vi "总磷总氮测量流程.vi"(8 "启动参数":cluster{"总磷":bool, "总氮":bool}={"总磷"=TRUE, "总氮"=TRUE}, 9 "总氮量程模式":T1, 10 "总磷量程模式":T1, 11 "参数":T2={"站号"=1, "量程切换"=enum."AUTO", "控制命令"=enum."启动测量", "模式设置"=enum."待机", "测量间隔"=0} {"站号" items=["总磷"=1, "总氮"=2]}) -> ()   [LabVIEW 2016, in "斯坦道总磷总氮.lvlib"]
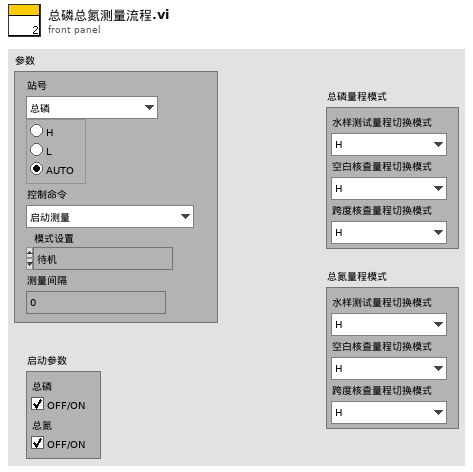
[diagram p1: front panel]
types:
  T1 = cluster{"水样测试量程切换模式":enum16{"H", "L", "AUTO"}, "空白核查量程切换模式":enum16{"H", "L", "AUTO"}, "跨度核查量程切换模式":enum16{"H", "L", "AUTO"}}
  T2 = cluster{"站号":u16, "量程切换":enum32{"H", "L", "AUTO"}, "控制命令":enum16{"启动测量", "标样核查", "零点核查", "跨度核查", "空白测试", "平行样测试", "加标回收", "空白校准", "标样校准", "初始化（清洗）", "停止测试", "仪器重启", "校时", "模式设置", "测量间隔设置"}, "模式设置":enum16{"待机", "连续模式", "周期模式", "定点模式", "受控模式", "手动模式"}, "测量间隔":u16}
  T3 = enum16{"初始化", "通电", "参数1启动", "等待参数1测试完成", "参数1测试完成", "参数1存储数据", "参数2启动", "等待参数2测试完成", "参数2测试完成", "参数2存储数据", "断电", "结束"}
  T4 = cluster{"运行模式":enum16{"维护模式", "常规模式", "应急模式", "质控模式"}, "质控频次":enum16{"关闭", "每天", "星期一", "星期二", "星期三", "星期四", "星期五", "星期六", "星期日"}, "空白核查时间":u16, "跨度核查时间":u16, "24H周期设置":bool[]}
  T5 = cluster{"时间标识":timestamp, "设备":string, "日志信息":string, "流程参数":string}
  T6 = cluster{"时间标识":timestamp, "监测值":sgl, "单位":u16, "数据标识":string, "因子编码":u32, "标样参考值":sgl, "F0":sgl, "F1":sgl, "F2":sgl, "F3":sgl, "F4":sgl, "F5":sgl, "F6":sgl, "F7":sgl, "X":sgl, "温度":sgl, "湿度":sgl, "量程标识":string}
  T7 = enum16{"维护数据", "水样测试", "标样核查", "零点核查", "跨度核查", "空白测试", "平行样测试", "加标回收", "空白校准", "标样校准", "初始化（清洗）"}
  T8 = enum16{"启动测量", "标样核查", "零点核查", "跨度核查", "空白测试", "平行样测试", "加标回收", "空白校准", "标样校准", "初始化（清洗）", "停止测试", "仪器重启", "校时", "模式设置", "测量间隔设置"}
  T9 = cluster{"系统时间":timestamp, "工作状态":enum16{"空闲", "水样测试", "标样核查", "零点核查", "跨度核查", "空白测试", "平行样测试", "加标回收", "空白校准", "标样校准", "初始化（清洗）"}, "测量模式":enum16{"待机", "连续模式", "周期模式", "定点模式", "受控模式", "手动模式"}, "告警代码":enum16{"无告警", "缺试剂告警", "缺水样告警", "缺蒸馏水告警", "缺标液告警", "仪表漏液告警", "标定异常告警", "超量程告警", "加热异常", "低试剂预警", "超上限告警", "超下限告警", "仪表内部其他异常", "滴定异常告警", "电极异常告警", "量程切换告警", "参数设置告警", "PH电极电位异常", "电导率电极异常", "浊度光度异常", "溶解氧电极异常", "溶解氧光强异常", "温度异常告警", "PH异常告警", "溶解氧异常告警", "电导率异常告警", "浊度异常告警", "叶绿素异常告警", "藻密度异常告警", "蓝绿藻异常告警", "ORP异常告警", "氨氮异常告警", "清洁刷异常告警", "SD卡异常告警", "蓝牙异常告警", "Wifi异常告警", "流程异常告警"}, "故障代码":enum16{"无故障", "电机故障", "温度故障", "通讯故障", "滴定故障"}, "日志代码":u16, "软件版本":u16, "F0":sgl, "F1":sgl, "F2":sgl, "F3":sgl, "T":sgl, "H":sgl, "id":u16, "flowid":u16, "量程":u16, "总磷控温温度1":sgl, "营养盐控温温度2":sgl, "ADC":sgl}
  T10 = enum16{"空闲", "水样测试", "标样核查", "零点核查", "跨度核查", "空白测试", "平行样测试", "加标回收", "空白校准", "标样校准", "初始化（清洗）"}
  T11 = cluster{"因子编码":u32, "单位":u16, "标样参考值":sgl, "水样数据时间":timestamp, "水样实测值":sgl, "水样数据标识":string, "标样数据时间":timestamp, "标样实测值":sgl, "标样数据标识":string, "空白数据时间":timestamp, "空白实测值":sgl, "空白数据标识":string, "零点核查数据时间":timestamp, "零点核查实测值":sgl, "零点核查数据标识":string, "跨度核查数据时间":timestamp, "跨度核查实测值":sgl, "跨度核查数据标识":string, "加标回收数据时间":timestamp, "加标回收实测值":sgl, "加标回收数据标识":string, "平行样数据时间":timestamp, "平行样实测值":sgl, "平行样数据标识":string, "F0":sgl, "F1":sgl, "F2":sgl, "F3":sgl, "F4":sgl, "F5":sgl, "F6":sgl, "F7":sgl, "温度":sgl, "湿度":sgl, "X值":sgl}
  T12 = cluster{"总磷跨度值":dbl, "总磷零点标准液浓度":dbl, "总磷跨度标准液浓度":dbl, "总磷标准液标准浓度":dbl, "总氮跨度值":dbl, "总氮零点标准液浓度":dbl, "总氮跨度标准液浓度":dbl, "总氮标准液标准浓度":dbl}
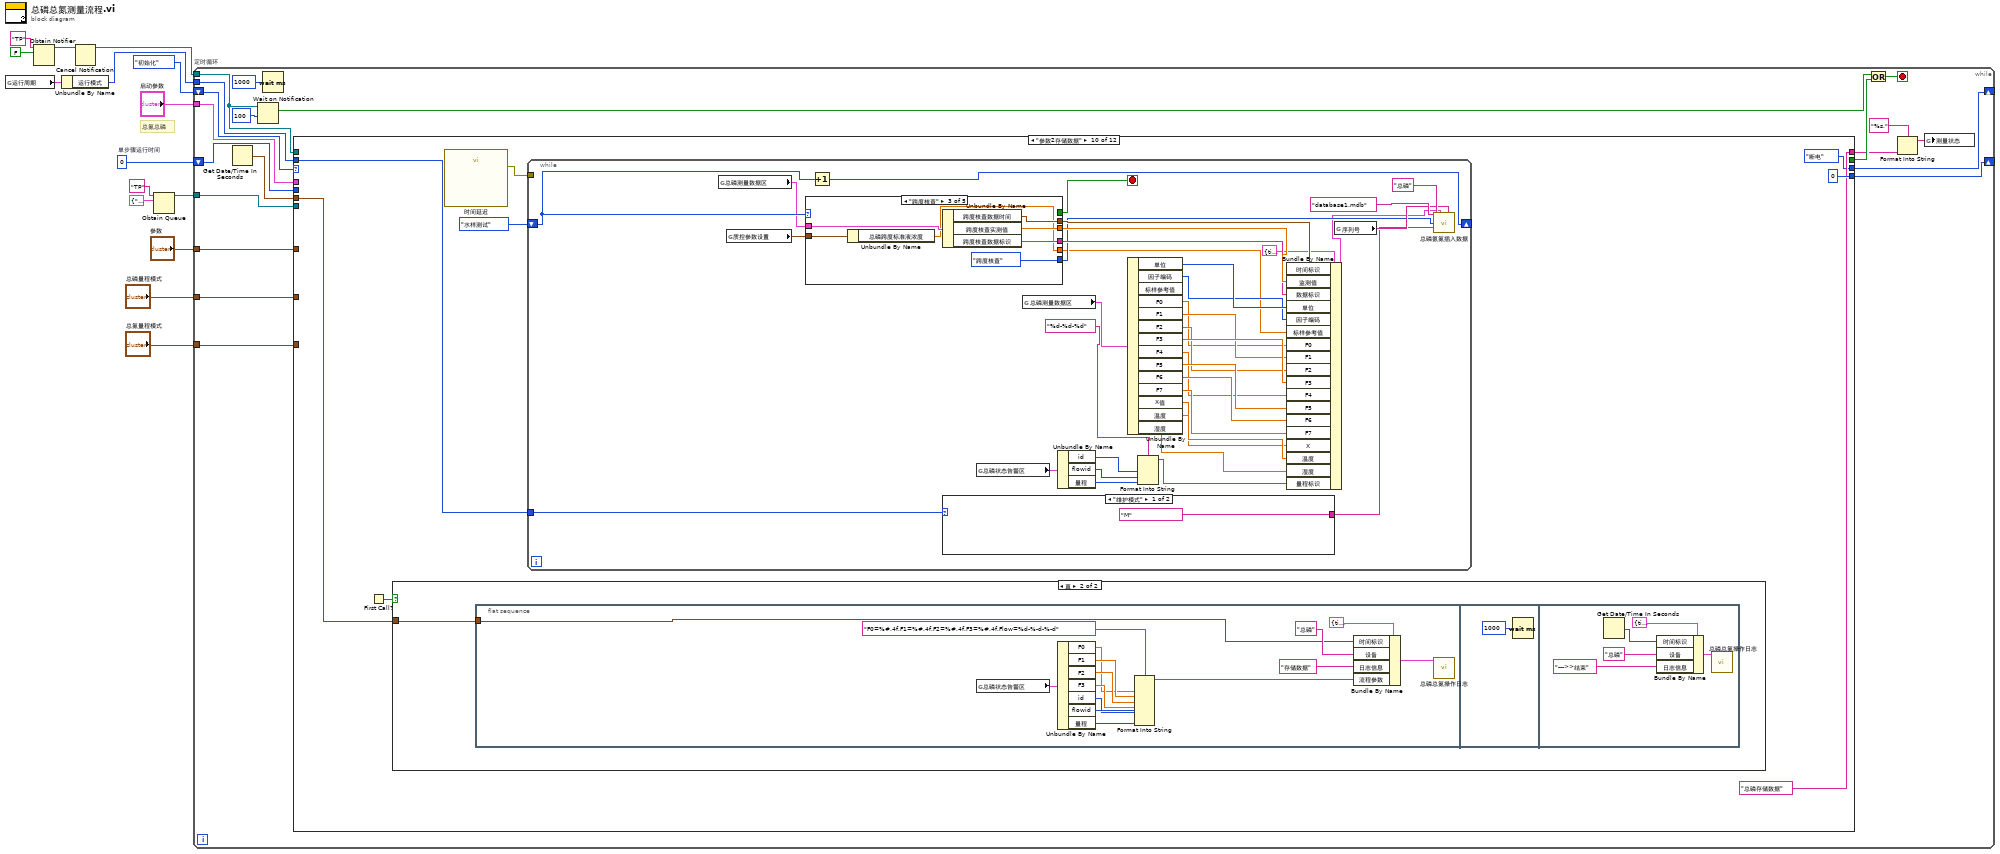
[diagram p0: block diagram]
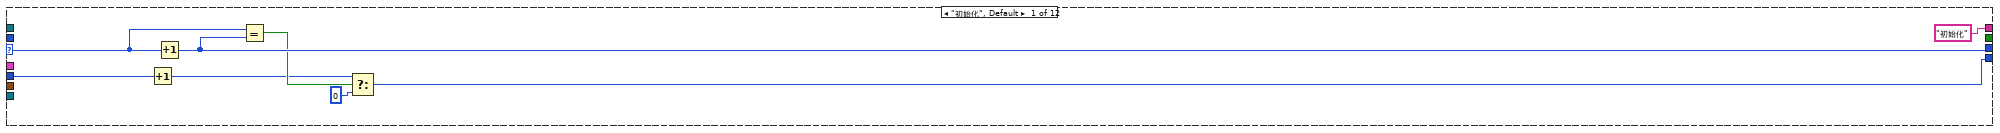
[diagram p2: hidden frame]
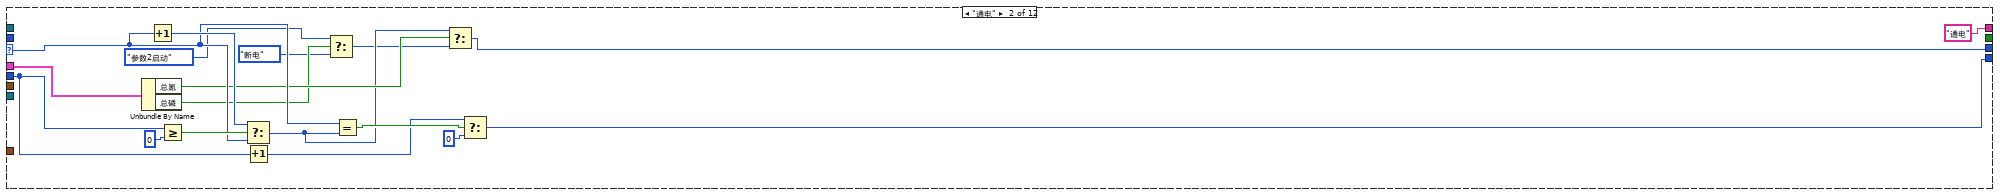
[diagram p3: hidden frame]
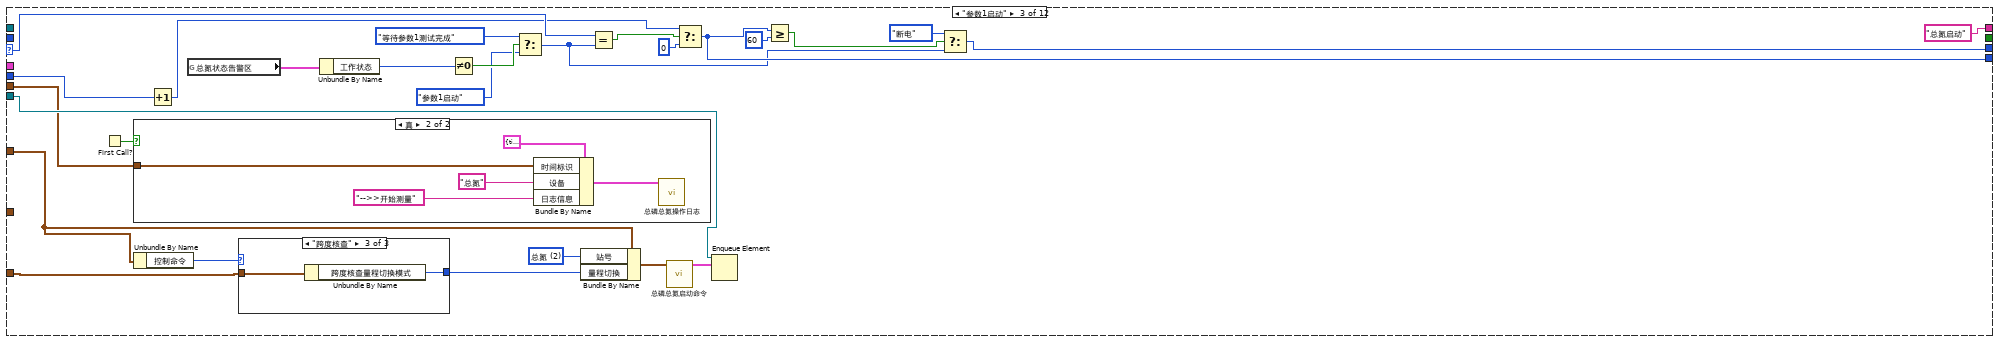
[diagram p4: hidden frame]
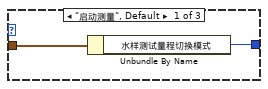
[diagram p5: hidden frame]
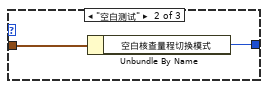
[diagram p6: hidden frame]
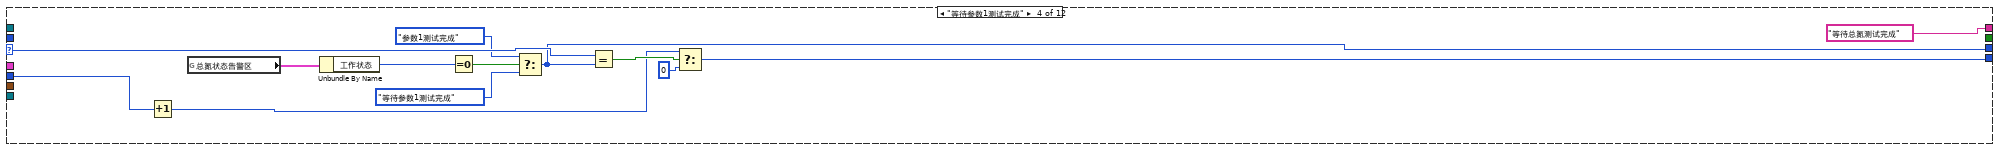
[diagram p8: hidden frame]
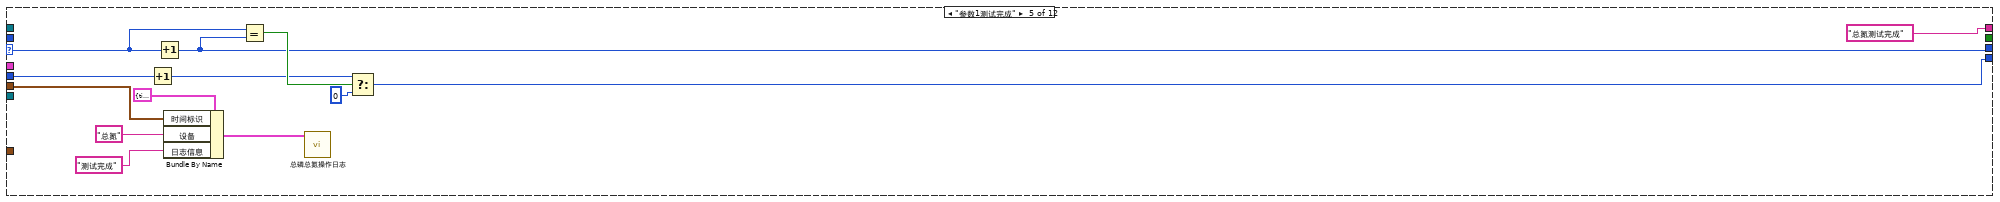
[diagram p9: hidden frame]
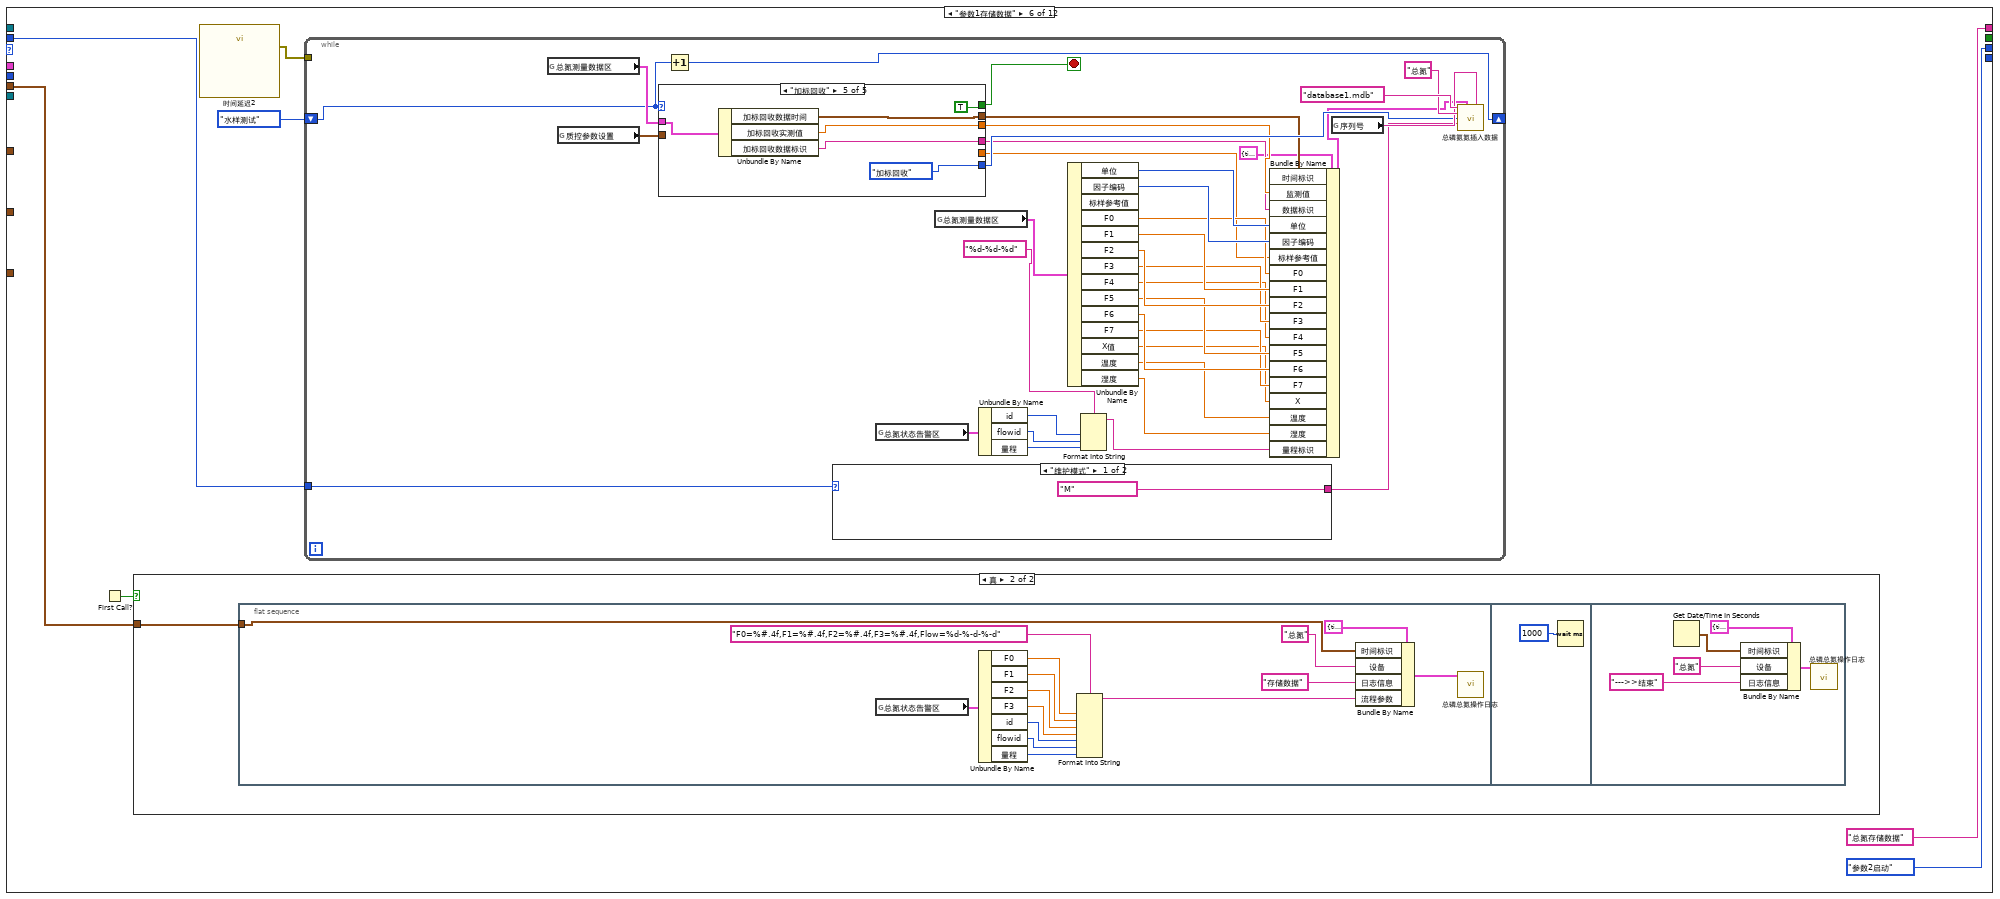
[diagram p10: hidden frame]
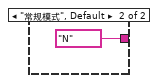
[diagram p11: hidden frame]
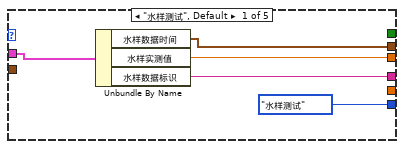
[diagram p12: hidden frame]
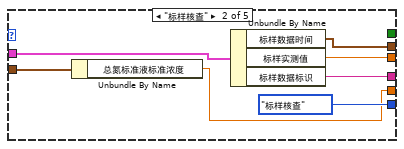
[diagram p13: hidden frame]
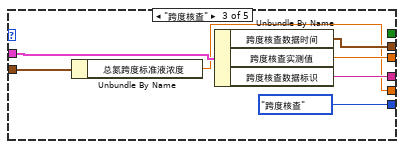
[diagram p14: hidden frame]
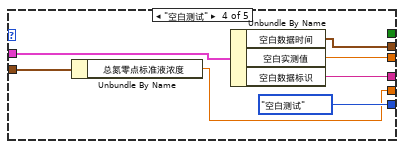
[diagram p15: hidden frame]
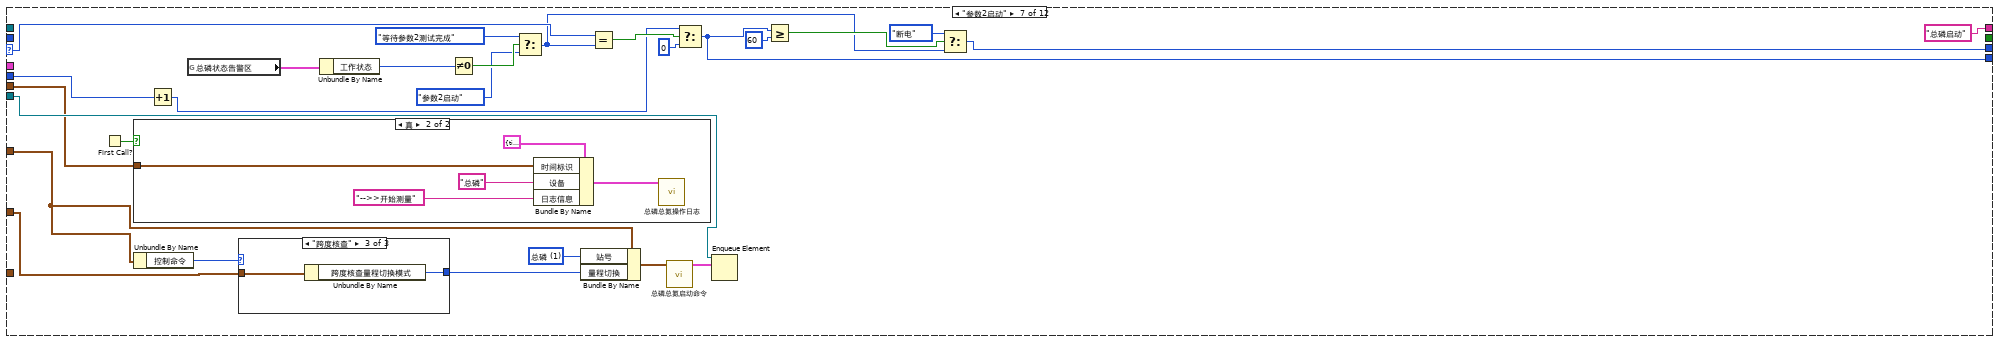
[diagram p17: hidden frame]
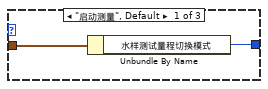
[diagram p18: hidden frame]
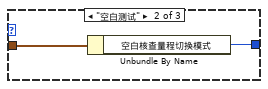
[diagram p19: hidden frame]
diagram:
  w11 = 0  # 单步骤运行时间
  # "总氮总磷"
  n1 = global read "总磷总氮断电保存全局变量.vi" "运行周期"() -> (w2:T4)
  n2 = Obtain Notifier(name (unnamed)="TP" ("名称（未命名）"), notification data type=FALSE) -> (notifier out=w8:refnum<notifier>)  [unwired: 2 in, 2 out]
  n3 = Unbundle By Name(w2) -> ("运行模式"=w1:enum16{"维护模式", "常规模式", "应急模式", "质控模式"})
  n4 = Cancel Notification(0:w8) -> (8:w7:refnum<notifier>)  [unwired: 1 in, 2 out]
  n5 = Obtain Queue(name (unnamed)="TP" ("名称（未命名）"), element data type=cluster{"命令":string, "data":variant} {"命令"="", "data"=variant}) -> (queue out=w12:refnum<queue>)  [unwired: 3 in, 2 out]
  n6 = while "定时循环" {
    shift-right: [w34] -> _
    shift-left: T3."初始化" ("枚举") -> [w35]
    tunnel: w12 -> [w33]
    shift-right: [w31] -> _
    shift-left: w11 -> [w32]
    tunnel: w7 -> [w30]
    tunnel: "参数" -> [w25]
    tunnel: "总氮量程模式" -> [w20]
    tunnel: "总磷量程模式" -> [w18]
    tunnel: "启动参数" -> [w17]
    tunnel: w1 -> [w16]
    stop <- w26 stop-if-true
    n7 = Get Date/Time In Seconds() -> (seconds since 1Jan1904=w23:timestamp)
    n8 = Wait on Notification(notifier=w30, timeout in ms (-1)=100 ("超时毫秒(-1)")) -> (notification=w27:bool)  [unwired: 2 in, 3 out]
    n9 = Wait (ms)(milliseconds to wait=u32 1000 ("等待时间（毫秒）")) -> ()  [unwired: 1 out]
    n10 = case shown="\"参数2存储数据\"" w35 {
      selector: w35 -> [w41 w55 w83 w107 w122 _ w241 w269 w285 _ w396 _]
      tunnel: [_ _ _ _ _ _ _ _ _ _ _ TRUE] -> w28
      tunnel: [w42 w48 w62 w106 w121 T3."参数2启动" ("枚举") w227 w267 w283 T3."断电" ("枚举") w395 T3."结束" ("枚举")] -> w34
      tunnel: w33 -> [_ _ w88 _ _ _ w249 _ _ _ _ w403]
      tunnel: w32 -> [w43 w56 w84 w109 w123 _ w242 w270 w286 _ w398 _]
      tunnel: [w39 w57 w67 w108 w124 _ w228 w268 w284 0 ("t") w397 0 ("t")] -> w31
      tunnel: w30 -> [_ _ _ _ _ _ _ _ _ _ _ w402]
      tunnel: w25 -> [_ _ w71 _ _ _ w235 _ _ _ _ _]
      tunnel: w23 -> [_ _ w76 _ w114 w132 w240 _ w278 w296 _ _]
      tunnel: ["初始化" ("输入 1") "通电" ("输入 1") "总氮启动" ("输入 1") "等待总氮测试完成" ("输入 1") "总氮测试完成" ("输入 1") "总氮存储数据" ("输入 1") "总磷启动" ("输入 1") "等待总磷测试完成" ("输入 1") "总磷测试完成" ("输入 1") "总磷存储数据" ("输入 1") "断电" ("输入 1") "结束" ("输入 1")] -> w21
      tunnel: w20 -> [_ _ w69 _ _ _ _ _ _ _ _ _]
      tunnel: w18 -> [_ _ _ _ _ _ w226 _ _ _ _ _]
      tunnel: w17 -> [_ w51 _ _ _ _ _ _ _ _ _ _]
      tunnel: w16 -> [_ _ _ _ _ w126 _ _ _ w290 _ _]
      frame "初始化", Default {
        n11 = Increment(x=w43) -> (x+1=w37:i32)
        n12 = Increment(x=w41) -> (x+1=w42:T3)
        n13 = Equal?(x=w41, y=w42) -> (x = y?=w40:bool)
        n14 = Select(t=w37, s=w40, f=0 ("t")) -> (s? t:f=w39:i32)
      }
      frame "通电" {
        n15 = Unbundle By Name(w51) -> ("总氮"=w50:bool, "总磷"=w47:bool)
        n16 = Increment(x=w55) -> (x+1=w59:T3)
        n17 = Greater Or Equal?(x=w56, y=0) -> (x >= y?=w60:bool)
        n18 = Select(t=w59, s=w60, f=w55) -> (s? t:f=w49:T3)
        n19 = Increment(x=w56) -> (x+1=w54:i32)
        n20 = Select(t=T3."参数2启动" ("枚举"), s=w47, f=T3."断电" ("枚举")) -> (s? t:f=w44:T3)
        n21 = Equal?(x=w55, y=w49) -> (x = y?=w58:bool)
        n22 = Select(t=w49, s=w50, f=w44) -> (s? t:f=w48:T3)
        n23 = Select(t=w54, s=w58, f=0 ("t")) -> (s? t:f=w57:i32)
      }
      frame "参数1启动" {
        w78 = u16 2 items=["总磷"=1, "总氮"=2, "氨氮"=3] ("站号")
        n24 = First Call?() -> (First Call?: T/F=w75:bool)
        n25 = case shown="真" w75 {
          tunnel: w76 -> [_ w95]
          frame False {
          }
          frame True {
            n26 = Bundle By Name(cluster=T5 {"时间标识"=timestamp(0 s since 1904-01-01), "设备"="", "日志信息"="", "流程参数"=""} ("data in"), "时间标识"=w95, "设备"="总氮", "日志信息"="-->>开始测量") -> (w99:T5)
            n27 = call "总磷总氮操作日志.vi"("data in"=w99) -> ()  [unwired: 11 in]
          }
        }
        n28 = Unbundle By Name(w71) -> ("控制命令"=w70:T8)
        n29 = Increment(x=w84) -> (x+1=w81:i32)
        n30 = global read "VAR总磷总氮全局变量.vi" "总氮状态告警区"() -> (w77:T9)
        n31 = case shown="\"跨度核查\"" w70 {
          tunnel: w69 -> [w90 w92 w94]
          tunnel: [w89 w91 w93] -> w68
          frame "启动测量", Default {
            n32 = Unbundle By Name(w90) -> ("水样测试量程切换模式"=w89:enum16{"H", "L", "AUTO"})
          }
          frame "空白测试" {
            n33 = Unbundle By Name(w92) -> ("空白核查量程切换模式"=w91:enum16{"H", "L", "AUTO"})
          }
          frame "跨度核查" {
            n34 = Unbundle By Name(w94) -> ("跨度核查量程切换模式"=w93:enum16{"H", "L", "AUTO"})
          }
        }
        n35 = Unbundle By Name(w77) -> ("工作状态"=w87:T10)
        n36 = Not Equal To 0?(x=w87) -> (x != 0?=w86:bool)
        n37 = Select(t=T3."等待参数1测试完成" ("枚举"), s=w86, f=T3."参数1启动" ("枚举")) -> (s? t:f=w64:T3)
        n38 = Bundle By Name(cluster=w71, "站号"=w78, "量程切换"=w68) -> (w79:T2)
        n39 = Equal?(x=w83, y=w64) -> (x = y?=w85:bool)
        n40 = call "总磷总氮启动命令.vi"("参数"=w79) -> ("启动命令"=w80:cluster{"命令":string, "data":variant})  [unwired: 10 in]
        n41 = Select(t=w81, s=w85, f=0 ("t")) -> (s? t:f=w67:i32)
        n42 = Enqueue Element(queue=w88, element=w80) -> ()  [unwired: 2 in, 3 out]
        n43 = Greater Or Equal?(x=w67, y=60) -> (x >= y?=w65:bool)
        n44 = Select(t=T3."断电" ("枚举"), s=w65, f=w64) -> (s? t:f=w62:T3)
      }
      frame "等待参数1测试完成" {
        n45 = Increment(x=w109) -> (x+1=w104:i32)
        n46 = global read "VAR总磷总氮全局变量.vi" "总氮状态告警区"() -> (w103:T9)
        n47 = Unbundle By Name(w103) -> ("工作状态"=w112:T10)
        n48 = Equal To 0?(x=w112) -> (x = 0?=w111:bool)
        n49 = Select(t=T3."参数1测试完成" ("枚举"), s=w111, f=T3."等待参数1测试完成" ("枚举")) -> (s? t:f=w106:T3)
        n50 = Equal?(x=w107, y=w106) -> (x = y?=w110:bool)
        n51 = Select(t=w104, s=w110, f=0 ("t")) -> (s? t:f=w108:i32)
      }
      frame "参数1测试完成" {
        n52 = Increment(x=w123) -> (x+1=w119:i32)
        n53 = Increment(x=w122) -> (x+1=w121:T3)
        n54 = Bundle By Name(cluster=T5 {"时间标识"=timestamp(0 s since 1904-01-01), "设备"="", "日志信息"="", "流程参数"=""} ("data in"), "时间标识"=w114, "设备"="总氮", "日志信息"="测试完成") -> (w118:T5)
        n55 = Equal?(x=w122, y=w121) -> (x = y?=w125:bool)
        n56 = call "总磷总氮操作日志.vi"("data in"=w118) -> ()  [unwired: 11 in]
        n57 = Select(t=w119, s=w125, f=0 ("t")) -> (s? t:f=w124:i32)
      }
      frame "参数1存储数据" {
        n58 = First Call?() -> (First Call?: T/F=w130:bool)
        n59 = case shown="真" w130 {
          tunnel: w132 -> [_ w204]
          frame False {
          }
          frame True {
            n60 = flat-sequence {
              tunnel: w204 -> [w215]
              frame #0 {
                n61 = global read "VAR总磷总氮全局变量.vi" "总氮状态告警区"() -> (w214:T9)
                n62 = Unbundle By Name(w214) -> ("F0"=w206:sgl, "F1"=w207:sgl, "F2"=w208:sgl, "F3"=w209:sgl, "id"=w210:u16, "flowid"=w211:u16, "量程"=w212:u16)
                n63 = Format Into String(format string="F0=%#.4f,F1=%#.4f,F2=%#.4f,F3=%#.4f,Flow=%d-%-d-%-d" ("格式字符串"), w206, w207, w208, w209, w210, w211, w212) -> (resulting string=w205:string)  [unwired: 2 in, 1 out]
                n64 = Bundle By Name(cluster=T5 {"时间标识"=timestamp(0 s since 1904-01-01), "设备"="", "日志信息"="", "流程参数"=""} ("data in"), "时间标识"=w215, "设备"="总氮", "日志信息"="存储数据", "流程参数"=w205) -> (w219:T5)
                n65 = call "总磷总氮操作日志.vi"("data in"=w219) -> ()  [unwired: 11 in]
              }
              frame #1 {
                n66 = Wait (ms)(milliseconds to wait=u32 1000 ("等待时间（毫秒）")) -> ()  [unwired: 1 out]
              }
              frame #2 {
                n67 = Get Date/Time In Seconds() -> (seconds since 1Jan1904=w221:timestamp)
                n68 = Bundle By Name(cluster=T5 {"时间标识"=timestamp(0 s since 1904-01-01), "设备"="", "日志信息"="", "流程参数"=""} ("data in"), "时间标识"=w221, "设备"="总氮", "日志信息"="--->>结束") -> (w222:T5)
                n69 = call "总磷总氮操作日志.vi"("data in"=w222) -> ()  [unwired: 11 in]
              }
            }
          }
        }
        n70 = call "时间延迟2"() -> ("error out"=w127:errorcluster)  [unwired: 11 in]
        n71 = while {
          shift-right: [w157] -> _
          shift-left: enum16{"水样测试", "标样核查", "跨度核查", "空白测试", "加标回收"}."水样测试" ("测量模式") -> [w158]
          tunnel: w127 -> [_]
          tunnel: w126 -> [w133]
          stop <- w159 stop-if-true
          n72 = global read "VAR总磷总氮全局变量.vi" "总氮测量数据区"() -> (w161:T11)
          n73 = global read "总磷总氮断电保存全局变量.vi" "质控参数设置"() -> (w136:T12)
          n74 = case shown="\"加标回收\"" w158 {
            tunnel: w161 -> [w172 w179 w186 w193 w198]
            tunnel: [w176 w183 w190 w197 w203] -> w155
            tunnel: [w175 w182 w189 w196 w202] -> w154
            tunnel: [w174 w181 w188 w195 w201] -> w153
            tunnel: [T7."水样测试" ("测量模式") T7."标样核查" ("测量模式") T7."跨度核查" ("测量模式") T7."空白测试" ("测量模式") T7."加标回收" ("测量模式")] -> w160
            tunnel: [_ _ _ _ TRUE] -> w159
            tunnel: w136 -> [_ w178 w185 w192 _]
            tunnel: [_ w177 w184 w191 _] -> w135
            frame "水样测试", Default {
              n75 = Unbundle By Name(w172) -> ("水样数据时间"=w176:timestamp, "水样实测值"=w175:sgl, "水样数据标识"=w174:string)
            }
            frame "标样核查" {
              n76 = Unbundle By Name(w178) -> ("总氮标准液标准浓度"=w177:dbl)
              n77 = Unbundle By Name(w179) -> ("标样数据时间"=w183:timestamp, "标样实测值"=w182:sgl, "标样数据标识"=w181:string)
            }
            frame "跨度核查" {
              n78 = Unbundle By Name(w185) -> ("总氮跨度标准液浓度"=w184:dbl)
              n79 = Unbundle By Name(w186) -> ("跨度核查数据时间"=w190:timestamp, "跨度核查实测值"=w189:sgl, "跨度核查数据标识"=w188:string)
            }
            frame "空白测试" {
              n80 = Unbundle By Name(w192) -> ("总氮零点标准液浓度"=w191:dbl)
              n81 = Unbundle By Name(w193) -> ("空白数据时间"=w197:timestamp, "空白实测值"=w196:sgl, "空白数据标识"=w195:string)
            }
            frame "加标回收" {
              n82 = Unbundle By Name(w198) -> ("加标回收数据时间"=w203:timestamp, "加标回收实测值"=w202:sgl, "加标回收数据标识"=w201:string)
            }
          }
          n83 = Increment(x=w158) -> (x+1=w157:enum16{"水样测试", "标样核查", "跨度核查", "空白测试", "加标回收"})
          n84 = case shown="\"维护模式\"" w133 {
            tunnel: ["M" ("数据标记表") "N" ("数据标记表")] -> w134
            frame "维护模式" {
            }
            frame "常规模式", Default {
            }
          }
          n85 = global read "VAR总磷总氮全局变量.vi" "总氮状态告警区"() -> (w169:T9)
          n86 = global read "VAR总磷总氮全局变量.vi" "总氮测量数据区"() -> (w156:T11)
          n87 = Unbundle By Name(w169) -> ("id"=w165:u16, "flowid"=w164:u16, "量程"=w163:u16)
          n88 = Unbundle By Name(w156) -> ("单位"=w152:u16, "因子编码"=w151:u32, "F0"=w147:sgl, "F1"=w146:sgl, "F2"=w145:sgl, "F3"=w144:sgl, "F4"=w143:sgl, "F5"=w142:sgl, "F6"=w141:sgl, "F7"=w140:sgl, "X值"=w139:sgl, "温度"=w138:sgl, "湿度"=w137:sgl)  [unwired: 1 out]
          n89 = Format Into String(format string="%d-%d-%d" ("格式字符串"), w165, w164, w163) -> (resulting string=w148:string)  [unwired: 2 in, 1 out]
          n90 = Bundle By Name(cluster=T6 {"时间标识"=timestamp(0 s since 1904-01-01), "监测值"=0.0, "单位"=0, "数据标识"="", "因子编码"=0, "标样参考值"=0.0, "F0"=0.0, "F1"=0.0, "F2"=0.0, "F3"=0.0, "F4"=0.0, "F5"=0.0, "F6"=0.0, "F7"=0.0, "X"=0.0, "温度"=0.0, "湿度"=0.0, "量程标识"=""} ("data"), "时间标识"=w155, "监测值"=w154, "数据标识"=w153, "单位"=w152, "因子编码"=w151, "标样参考值"=w135, "F0"=w147, "F1"=w146, "F2"=w145, "F3"=w144, "F4"=w143, "F5"=w142, "F6"=w141, "F7"=w140, "X"=w139, "温度"=w138, "湿度"=w137, "量程标识"=w148) -> (w149:T6)
          n91 = global read "VAR总磷总氮全局变量.vi" "序列号"() -> (w162:string)
          n92 = call "总磷氨氮插入数据.vi"("database"="database1.mdb", "data"=w149, "SN"=w162, "table"="总氮", "测量模式"=w160, "数据标记表"=w134) -> ()  [unwired: 9 in, 1 out]
        }
      }
      frame "参数2启动" {
        w250 = u16 1 items=["总氮"=2, "总磷"=1] ("站号")
        n93 = First Call?() -> (First Call?: T/F=w239:bool)
        n94 = case shown="真" w239 {
          tunnel: w240 -> [_ w262]
          frame False {
          }
          frame True {
            n95 = Bundle By Name(cluster=T5 {"时间标识"=timestamp(0 s since 1904-01-01), "设备"="", "日志信息"="", "流程参数"=""} ("data in"), "时间标识"=w262, "设备"="总磷", "日志信息"="-->>开始测量") -> (w263:T5)
            n96 = call "总磷总氮操作日志.vi"("data in"=w263) -> ()  [unwired: 11 in]
          }
        }
        n97 = Unbundle By Name(w235) -> ("控制命令"=w234:T8)
        n98 = Increment(x=w242) -> (x+1=w244:i32)
        n99 = global read "VAR总磷总氮全局变量.vi" "总磷状态告警区"() -> (w243:T9)
        n100 = case shown="\"跨度核查\"" w234 {
          tunnel: w226 -> [w254 w256 w258]
          tunnel: [w253 w255 w257] -> w233
          frame "启动测量", Default {
            n101 = Unbundle By Name(w254) -> ("水样测试量程切换模式"=w253:enum16{"H", "L", "AUTO"})
          }
          frame "空白测试" {
            n102 = Unbundle By Name(w256) -> ("空白核查量程切换模式"=w255:enum16{"H", "L", "AUTO"})
          }
          frame "跨度核查" {
            n103 = Unbundle By Name(w258) -> ("跨度核查量程切换模式"=w257:enum16{"H", "L", "AUTO"})
          }
        }
        n104 = Unbundle By Name(w243) -> ("工作状态"=w248:T10)
        n105 = Not Equal To 0?(x=w248) -> (x != 0?=w247:bool)
        n106 = Select(t=T3."等待参数2测试完成" ("枚举"), s=w247, f=T3."参数2启动" ("枚举")) -> (s? t:f=w229:T3)
        n107 = Bundle By Name(cluster=w235, "站号"=w250, "量程切换"=w233) -> (w251:T2)
        n108 = Equal?(x=w241, y=w229) -> (x = y?=w246:bool)
        n109 = call "总磷总氮启动命令.vi"("参数"=w251) -> ("启动命令"=w252:cluster{"命令":string, "data":variant})  [unwired: 10 in]
        n110 = Select(t=w244, s=w246, f=0 ("t")) -> (s? t:f=w228:i32)
        n111 = Enqueue Element(queue=w249, element=w252) -> ()  [unwired: 2 in, 3 out]
        n112 = Greater Or Equal?(x=w228, y=60) -> (x >= y?=w231:bool)
        n113 = Select(t=T3."断电" ("枚举"), s=w231, f=w229) -> (s? t:f=w227:T3)
      }
      frame "等待参数2测试完成" {
        n114 = Increment(x=w270) -> (x+1=w272:i32)
        n115 = global read "VAR总磷总氮全局变量.vi" "总磷状态告警区"() -> (w271:T9)
        n116 = Unbundle By Name(w271) -> ("工作状态"=w276:T10)
        n117 = Equal To 0?(x=w276) -> (x = 0?=w275:bool)
        n118 = Select(t=T3."参数2测试完成" ("枚举"), s=w275, f=T3."等待参数2测试完成" ("枚举")) -> (s? t:f=w267:T3)
        n119 = Equal?(x=w269, y=w267) -> (x = y?=w274:bool)
        n120 = Select(t=w272, s=w274, f=0 ("t")) -> (s? t:f=w268:i32)
      }
      frame "参数2测试完成" {
        n121 = Increment(x=w286) -> (x+1=w287:i32)
        n122 = Increment(x=w285) -> (x+1=w283:T3)
        n123 = Bundle By Name(cluster=T5 {"时间标识"=timestamp(0 s since 1904-01-01), "设备"="", "日志信息"="", "流程参数"=""} ("data in"), "时间标识"=w278, "设备"="总磷", "日志信息"="测试完成") -> (w282:T5)
        n124 = Equal?(x=w285, y=w283) -> (x = y?=w289:bool)
        n125 = call "总磷总氮操作日志.vi"("data in"=w282) -> ()  [unwired: 11 in]
        n126 = Select(t=w287, s=w289, f=0 ("t")) -> (s? t:f=w284:i32)
      }
      frame "参数2存储数据" {
        n127 = First Call?() -> (First Call?: T/F=w293:bool)
        n128 = case shown="真" w293 {
          tunnel: w296 -> [_ w369]
          frame False {
          }
          frame True {
            n129 = flat-sequence {
              tunnel: w369 -> [w380]
              frame #0 {
                n130 = global read "VAR总磷总氮全局变量.vi" "总磷状态告警区"() -> (w379:T9)
                n131 = Unbundle By Name(w379) -> ("F0"=w371:sgl, "F1"=w372:sgl, "F2"=w373:sgl, "F3"=w374:sgl, "id"=w375:u16, "flowid"=w376:u16, "量程"=w377:u16)
                n132 = Format Into String(format string="F0=%#.4f,F1=%#.4f,F2=%#.4f,F3=%#.4f,Flow=%d-%-d-%-d" ("格式字符串"), w371, w372, w373, w374, w375, w376, w377) -> (resulting string=w370:string)  [unwired: 2 in, 1 out]
                n133 = Bundle By Name(cluster=T5 {"时间标识"=timestamp(0 s since 1904-01-01), "设备"="", "日志信息"="", "流程参数"=""} ("data in"), "时间标识"=w380, "设备"="总磷", "日志信息"="存储数据", "流程参数"=w370) -> (w384:T5)
                n134 = call "总磷总氮操作日志.vi"("data in"=w384) -> ()  [unwired: 11 in]
              }
              frame #1 {
                n135 = Wait (ms)(milliseconds to wait=u32 1000 ("等待时间（毫秒）")) -> ()  [unwired: 1 out]
              }
              frame #2 {
                n136 = Get Date/Time In Seconds() -> (seconds since 1Jan1904=w386:timestamp)
                n137 = Bundle By Name(cluster=T5 {"时间标识"=timestamp(0 s since 1904-01-01), "设备"="", "日志信息"="", "流程参数"=""} ("data in"), "时间标识"=w386, "设备"="总磷", "日志信息"="--->>结束") -> (w390:T5)
                n138 = call "总磷总氮操作日志.vi"("data in"=w390) -> ()  [unwired: 11 in]
              }
            }
          }
        }
        n139 = call "时间延迟"() -> ("error out"=w291:errorcluster)  [unwired: 11 in]
        n140 = while {
          shift-right: [w318] -> _
          shift-left: enum16{"水样测试", "标样核查", "跨度核查", "空白测试", "加标回收"}."水样测试" ("测量模式") -> [w319]
          tunnel: w291 -> [_]
          tunnel: w290 -> [w298]
          stop <- w320 stop-if-true
          n141 = global read "VAR总磷总氮全局变量.vi" "总磷测量数据区"() -> (w317:T11)
          n142 = global read "总磷总氮断电保存全局变量.vi" "质控参数设置"() -> (w300:T12)
          n143 = case shown="\"跨度核查\"" w319 {
            tunnel: w317 -> [w341 w348 w355 w362 w368]
            tunnel: [w340 w347 w354 w361 w367] -> w324
            tunnel: [w339 w346 w353 w360 w366] -> w323
            tunnel: [w338 w345 w352 w359 w365] -> w322
            tunnel: [T7."水样测试" ("测量模式") T7."标样核查" ("测量模式") T7."跨度核查" ("测量模式") T7."空白测试" ("测量模式") T7."加标回收" ("测量模式")] -> w321
            tunnel: [_ _ _ _ TRUE] -> w320
            tunnel: w300 -> [_ w343 w350 w357 _]
            tunnel: [_ w342 w349 w356 _] -> w299
            frame "水样测试", Default {
              n144 = Unbundle By Name(w341) -> ("水样数据时间"=w340:timestamp, "水样实测值"=w339:sgl, "水样数据标识"=w338:string)
            }
            frame "标样核查" {
              n145 = Unbundle By Name(w343) -> ("总磷标准液标准浓度"=w342:dbl)
              n146 = Unbundle By Name(w348) -> ("标样数据时间"=w347:timestamp, "标样实测值"=w346:sgl, "标样数据标识"=w345:string)
            }
            frame "跨度核查" {
              n147 = Unbundle By Name(w350) -> ("总磷跨度标准液浓度"=w349:dbl)
              n148 = Unbundle By Name(w355) -> ("跨度核查数据时间"=w354:timestamp, "跨度核查实测值"=w353:sgl, "跨度核查数据标识"=w352:string)
            }
            frame "空白测试" {
              n149 = Unbundle By Name(w357) -> ("总磷零点标准液浓度"=w356:dbl)
              n150 = Unbundle By Name(w362) -> ("空白数据时间"=w361:timestamp, "空白实测值"=w360:sgl, "空白数据标识"=w359:string)
            }
            frame "加标回收" {
              n151 = Unbundle By Name(w368) -> ("加标回收数据时间"=w367:timestamp, "加标回收实测值"=w366:sgl, "加标回收数据标识"=w365:string)
            }
          }
          n152 = Increment(x=w319) -> (x+1=w318:enum16{"水样测试", "标样核查", "跨度核查", "空白测试", "加标回收"})
          n153 = case shown="\"维护模式\"" w298 {
            tunnel: ["M" ("数据标记表") "N" ("数据标记表")] -> w301
            frame "维护模式" {
            }
            frame "常规模式", Default {
            }
          }
          n154 = global read "VAR总磷总氮全局变量.vi" "总磷状态告警区"() -> (w332:T9)
          n155 = global read "VAR总磷总氮全局变量.vi" "总磷测量数据区"() -> (w316:T11)
          n156 = Unbundle By Name(w332) -> ("id"=w328:u16, "flowid"=w327:u16, "量程"=w326:u16)
          n157 = Unbundle By Name(w316) -> ("单位"=w334:u16, "因子编码"=w333:u32, "F0"=w302:sgl, "F1"=w303:sgl, "F2"=w304:sgl, "F3"=w305:sgl, "F4"=w306:sgl, "F5"=w307:sgl, "F6"=w308:sgl, "F7"=w309:sgl, "X值"=w310:sgl, "温度"=w311:sgl, "湿度"=w312:sgl)  [unwired: 1 out]
          n158 = Format Into String(format string="%d-%d-%d" ("格式字符串"), w328, w327, w326) -> (resulting string=w313:string)  [unwired: 2 in, 1 out]
          n159 = Bundle By Name(cluster=T6 {"时间标识"=timestamp(0 s since 1904-01-01), "监测值"=0.0, "单位"=0, "数据标识"="", "因子编码"=0, "标样参考值"=0.0, "F0"=0.0, "F1"=0.0, "F2"=0.0, "F3"=0.0, "F4"=0.0, "F5"=0.0, "F6"=0.0, "F7"=0.0, "X"=0.0, "温度"=0.0, "湿度"=0.0, "量程标识"=""} ("data"), "时间标识"=w324, "监测值"=w323, "数据标识"=w322, "单位"=w334, "因子编码"=w333, "标样参考值"=w299, "F0"=w302, "F1"=w303, "F2"=w304, "F3"=w305, "F4"=w306, "F5"=w307, "F6"=w308, "F7"=w309, "X"=w310, "温度"=w311, "湿度"=w312, "量程标识"=w313) -> (w315:T6)
          n160 = global read "VAR总磷总氮全局变量.vi" "序列号"() -> (w325:string)
          n161 = call "总磷氨氮插入数据.vi"("database"="database1.mdb", "data"=w315, "SN"=w325, "table"="总磷", "测量模式"=w321, "数据标记表"=w301) -> ()  [unwired: 9 in, 1 out]
        }
      }
      frame "断电" {
        n162 = Increment(x=w398) -> (x+1=w391:i32)
        n163 = Increment(x=w396) -> (x+1=w395:T3)
        n164 = Equal?(x=w396, y=w395) -> (x = y?=w393:bool)
        n165 = Select(t=w391, s=w393, f=0 ("t")) -> (s? t:f=w397:i32)
      }
      frame "结束" {
        n166 = Release Queue(queue=w403) -> ()  [unwired: 2 in, 3 out]
        n167 = Cancel Notification(0:w402) -> (8:w401:refnum<notifier>)  [unwired: 1 in, 2 out]
        n168 = Release Notifier(notifier=w401) -> ()  [unwired: 2 in, 3 out]
      }
    }
    n169 = Or(x=w27, y=w28) -> (x .or. y?=w26:bool)
    n170 = Format Into String(format string="%s," ("格式字符串"), w21) -> (resulting string=w19:string)  [unwired: 2 in, 1 out]
    n171 = global write "VAR总磷总氮全局变量.vi" "测量状态"(w19) -> ()
  }
